vi "Item Properties.vi"(0 "Tree Reference In":refnum<vi>, 1 "Tag (Current)":string, 5 "error in (no error)":errorcluster, 9 "Column # (0)":i32) -> (11 "Cell String":string, 13 "Symbol Index":i32, 14 "Tree Reference Out":refnum<vi>, 15 "Duplicate Tag":string, 16 "Open?":bool, 17 "Child-Only?":bool, 18 "Indent Level":i32, 19 "error out":errorcluster)   [LabVIEW 2015, in "QuickVIew.lvlib"]
doc: "Gets a limited set of properties about the input item \nTLB Prime - Application Template 1.3.0.24\nNorm Kirchner, NI Systems Engineering - NI\nCopyright (c) 2014, NI"
uses:
  QuickVIew.lvlib
panel:
  # "VI INPUTS"
  # "VI OUTPUTS"
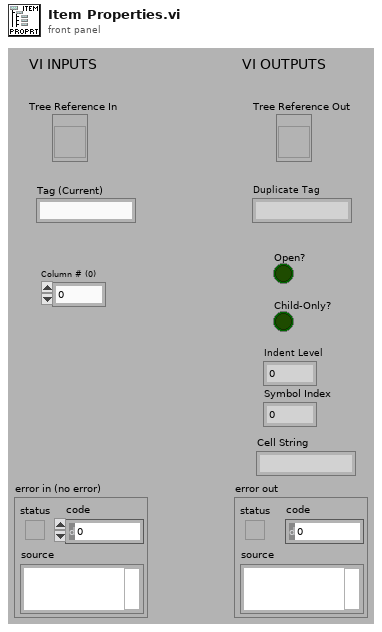
[diagram p1: front panel]
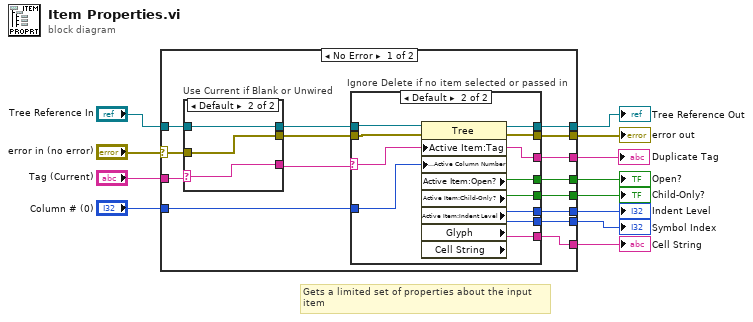
[diagram p0: block diagram]
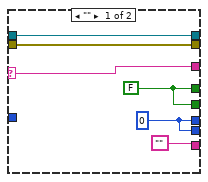
[diagram p2: hidden frame]
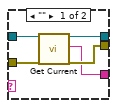
[diagram p3: hidden frame]
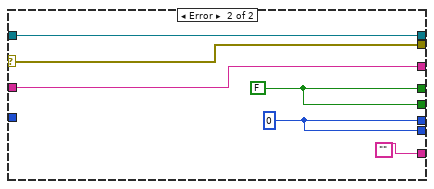
[diagram p4: hidden frame]
diagram:
  # "Gets a limited set of properties about the input item"
  n1 = case shown="No Error" "error in (no error)" {
    selector: "error in (no error)" -> [w25 w57]
    tunnel: "Tree Reference In" -> [w27 w58]
    tunnel: [w24 w58] -> w11
    tunnel: [w23 w57] -> w10
    tunnel: "Tag (Current)" -> [w26 w55]
    tunnel: "Column # (0)" -> [w19 _]
    tunnel: [w18 w56] -> w6
    tunnel: [w17 w56] -> w5
    tunnel: [w16 w54] -> w4
    tunnel: [w15 w55] -> w3
    tunnel: [w14 w54] -> w2
    tunnel: [w13 ""] -> w1
    frame No Error {
      n2 = case "Use Current if Blank or Unwired" shown="Default" w26 {
        selector: w26 -> [_ w50]
        tunnel: [w48 w52] -> w22
        tunnel: w27 -> [w49 w52]
        tunnel: [w47 w51] -> w21
        tunnel: w25 -> [w46 w51]
        tunnel: [w45 w50] -> w20
        frame "" {
          n3 = call "Get Current.vi"("Tree Reference In"=w49, "error in (no error)"=w46) -> ("Tree Reference Out"=w48:refnum<vi>, "Current Tag"=w45:string, "error out"=w47:errorcluster)  [unwired: 15 out]
        }
        frame Default {
        }
      }
      n4 = case "Ignore Delete if no item selected or passed in" shown="Default" w20 {
        selector: w20 -> [w30 w36]
        tunnel: [w33 w38] -> w24
        tunnel: [w32 w37] -> w23
        tunnel: w22 -> [w33 w44]
        tunnel: w21 -> [w32 w43]
        tunnel: w19 -> [_ w42]
        tunnel: [w31 w41] -> w18
        tunnel: [w31 w40] -> w17
        tunnel: [w29 w39] -> w16
        tunnel: [w30 w36] -> w15
        tunnel: [w29 w35] -> w14
        tunnel: ["" w34] -> w13
        frame "" {
          w29 = 0 ("Indent Level")
          w31 = FALSE ("Open?")
        }
        frame Default {
          n5 = property class="Tree"(reference=w44, error in=w43, "Active Item:Tag"=w36, "Active Cell:Active Column Number"=w42) -> (reference out=w38:refnum<vi>, error out=w37:errorcluster, "Active Item:Open?"=w41:bool, "Active Item:Child-Only?"=w40:bool, "Active Item:Indent Level"=w39:i32, "Glyph"=w35:i32, "Cell String"=w34:string)
        }
      }
    }
    frame Error {
      w54 = 0 ("Indent Level")
      w56 = FALSE ("Open?")
    }
  }
  "Tree Reference Out" <- w11
  "error out" <- w10
  "Open?" <- w6
  "Child-Only?" <- w5
  "Indent Level" <- w4
  "Duplicate Tag" <- w3
  "Symbol Index" <- w2
  "Cell String" <- w1
